vi "period.vi"() -> (3 ".":u8)   [LabVIEW 2021, in "d22.lvlib"]
uses:
  d22.lvlib
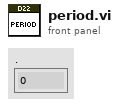
[diagram p1: front panel]
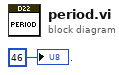
[diagram p0: block diagram]
diagram:
  "." <- u8 46 ("element")
